vi "HMI.vi"(5 "Disabled?":bool=TRUE, 7 "HMI to Control":T1={"RightDriveValue"=0.0, "LeftDriveValue"=0.0, "Arm Manual "=0.0, "Stacker Manual "=0.0, "Claw Manual "=0.0, "ClawSlightOpenNumber"=0, "Intake Value "=0.0, "Arm States"=enum."4 Tote", "Claw States"=enum."Claw Manual ", "Intake Man. or Sense"=enum."Sensing", "Stacker in Manual?"=FALSE, "Drop Stack? "=FALSE, "Tusk Up Request"=FALSE, "Tusk Down Request"=FALSE, "Inver. Wheels  In Request"=FALSE, "Inverse. Wheels Out Request "=FALSE, "Get Out of Manual Control"=FALSE, "Exit Score State"=FALSE, "DriveStraight Help?"=FALSE, "Stacker Shut Off No."=0, "Stacker Need Off?"=FALSE, "Collecting?"=FALSE, "Go to Hover"=FALSE, "Stack Clamp Lock "=FALSE, "Stack Clamp Unlock "=FALSE, "Claw Intake Value "=0.0, "Stack Clamp Lock No. "=0, "Steal Can (ruin their day?)"=FALSE, "Retract (have mercy?)"=FALSE, "Can Grab No. "=0, "Wench Value to Control "=0.0}, 9 "GamepadData":T5) -> (1 "HMI to Control Out":T1={"RightDriveValue"=0.0, "LeftDriveValue"=0.0, "Arm Manual "=0.0, "Stacker Manual "=0.0, "Claw Manual "=0.0, "ClawSlightOpenNumber"=0, "Intake Value "=0.0, "Arm States"=enum."4 Tote", "Claw States"=enum."Claw Manual ", "Intake Man. or Sense"=enum."Sensing", "Stacker in Manual?"=FALSE, "Drop Stack? "=FALSE, "Tusk Up Request"=FALSE, "Tusk Down Request"=FALSE, "Inver. Wheels  In Request"=FALSE, "Inverse. Wheels Out Request "=FALSE, "Get Out of Manual Control"=FALSE, "Exit Score State"=FALSE, "DriveStraight Help?"=FALSE, "Stacker Shut Off No."=0, "Stacker Need Off?"=FALSE, "Collecting?"=FALSE, "Go to Hover"=FALSE, "Stack Clamp Lock "=FALSE, "Stack Clamp Unlock "=FALSE, "Claw Intake Value "=0.0, "Stack Clamp Lock No. "=0, "Steal Can (ruin their day?)"=FALSE, "Retract (have mercy?)"=FALSE, "Can Grab No. "=0, "Wench Value to Control "=0.0}, 3 "GamepadDataOut":T5)   [LabVIEW 2014]
uses:
  Typedefs/GamepadData.ctl
  Typedefs/HMI_to_Control.ctl
  Typedefs/Arm States.ctl
  Typedefs/ClawStates.ctl
  Typedefs/IntakeWheelSenseOrManual.ctl
  Auton/scriptlib/auto_data.vi
panel:
  in  "Wheel Ramp Step":dbl=1.0 format="%#_13g"
  in  "Throttle Ramp Step":dbl=0.015
  in  "Claw Man Threshold":dbl=0.2
  in  "Throttle Drive Straight Assist Threshold":dbl=0.2
  in  "Wheel Drive Straight Assist Threshold":dbl=0.15
  in  "Man Threshold":dbl=0.3
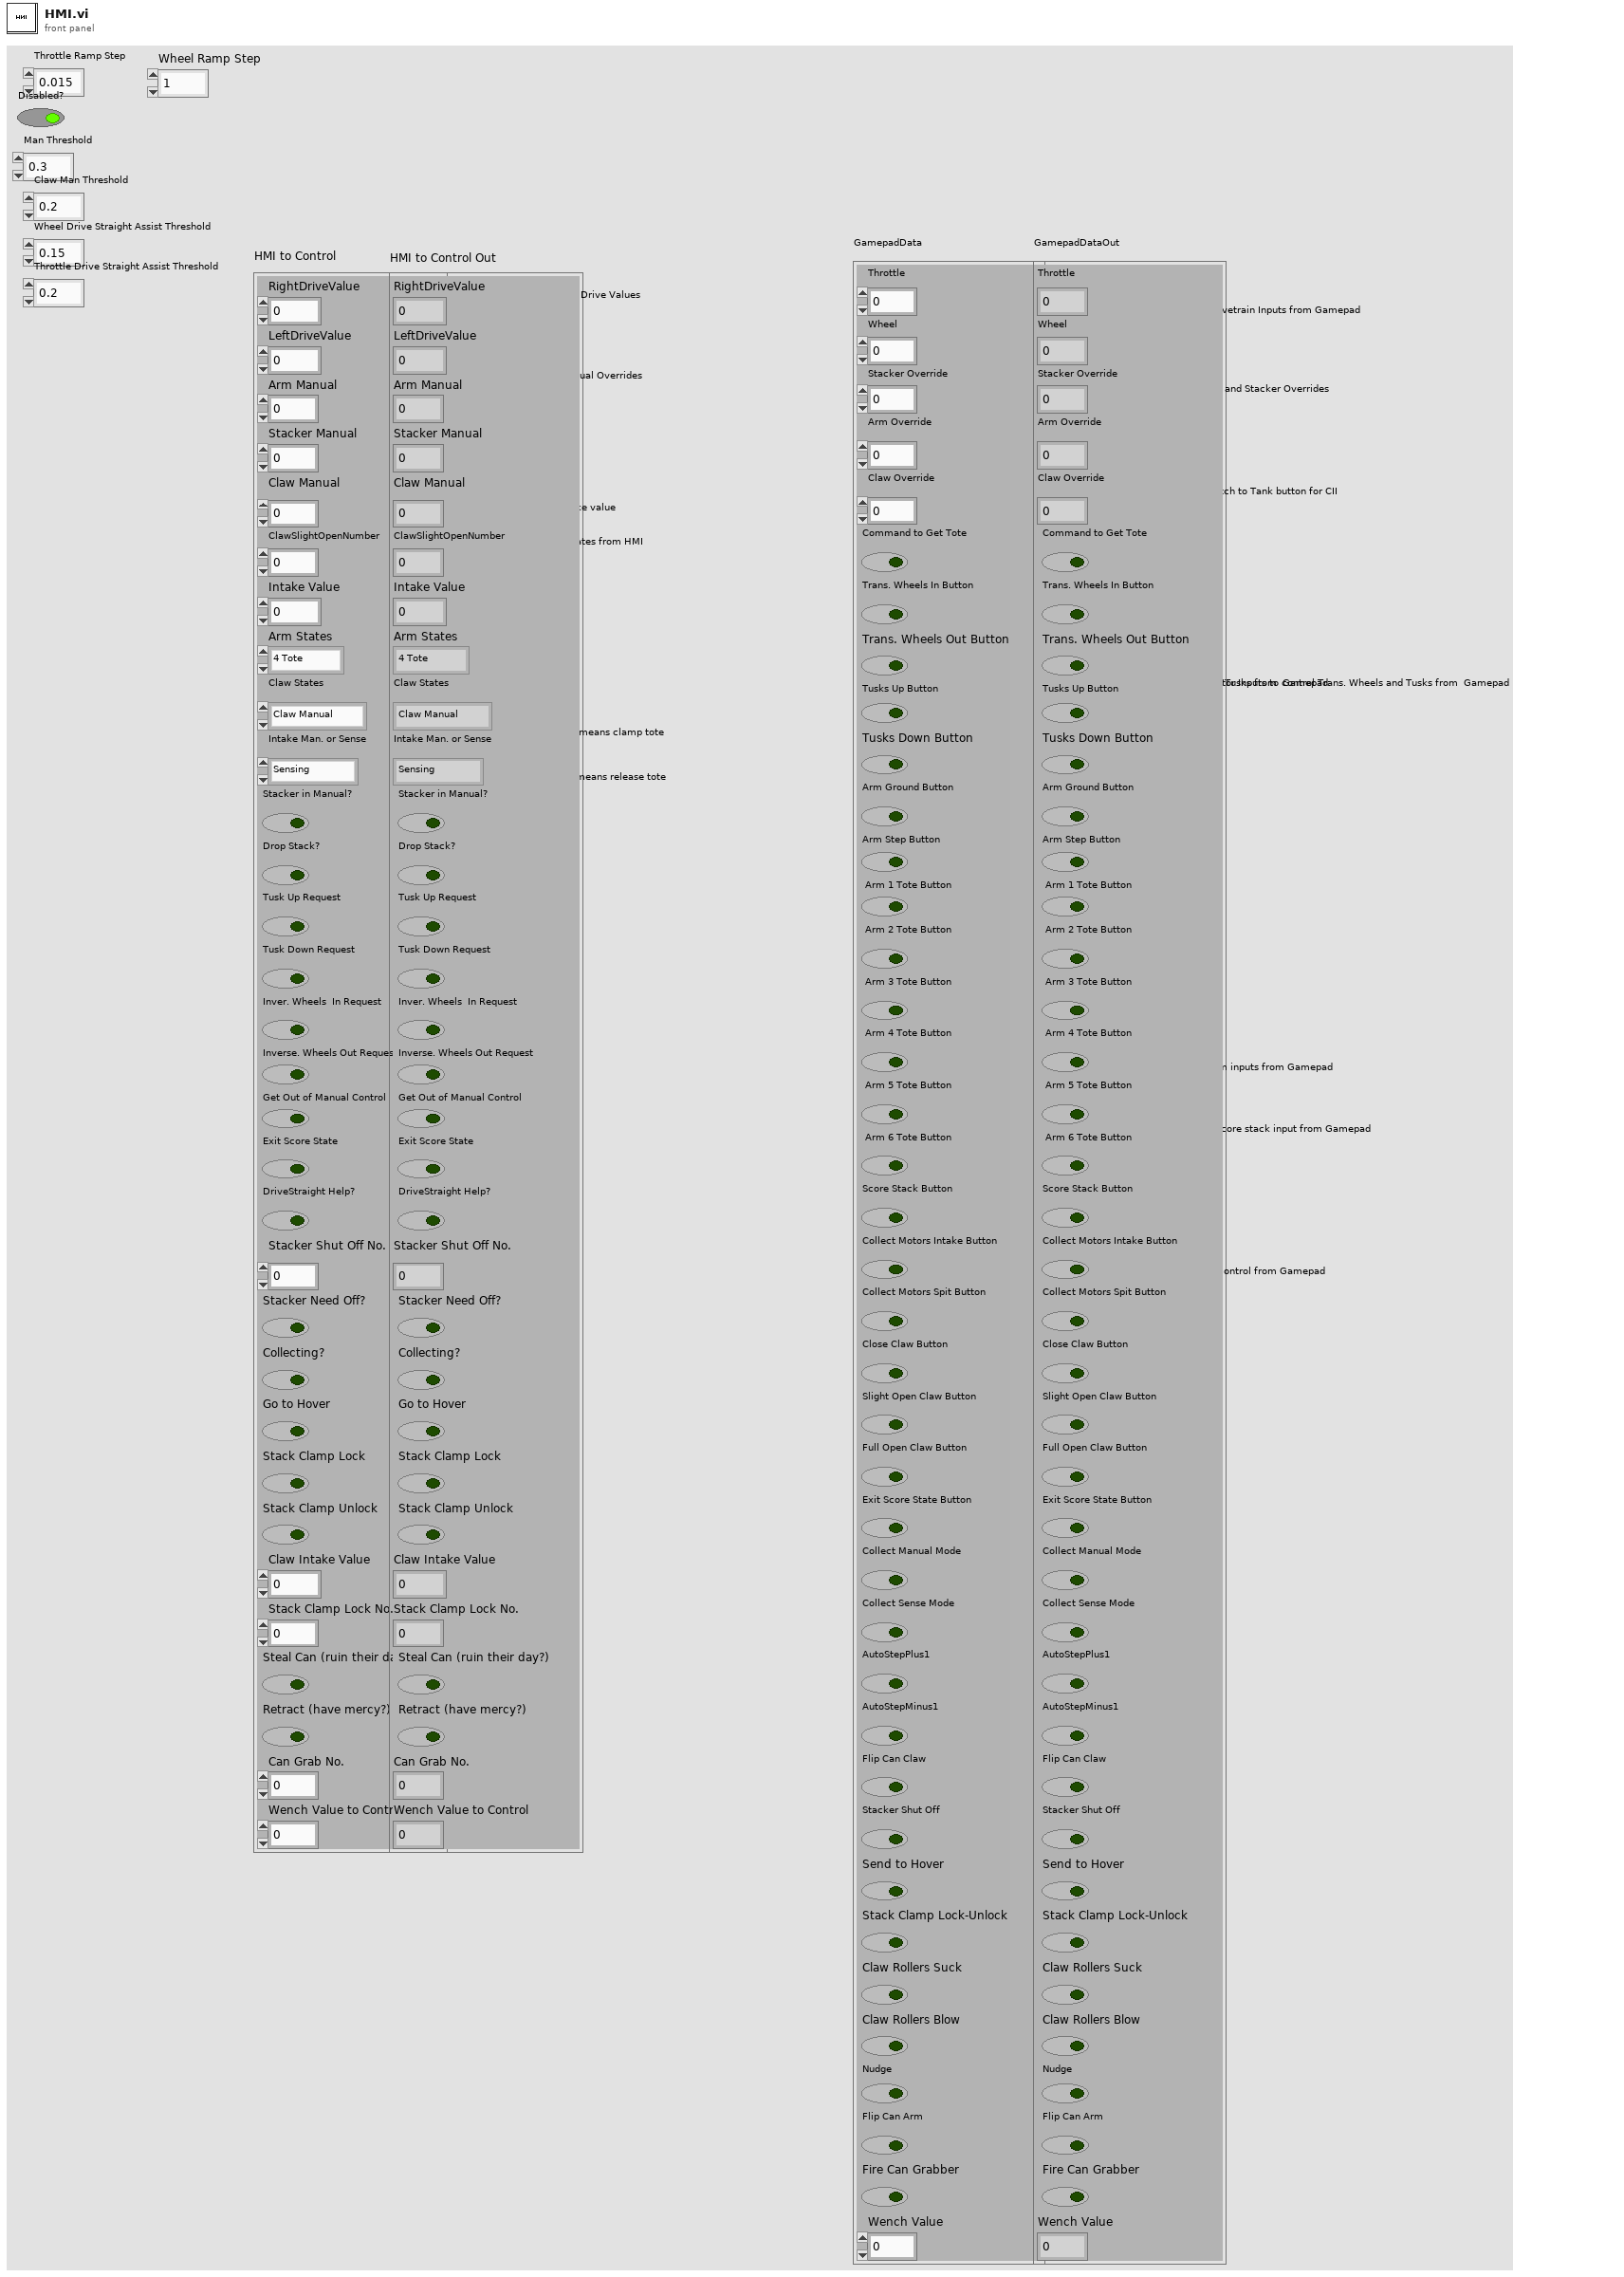
[diagram p1: front panel]
types:
  T1 = typedef "HMI_to_Control.ctl" = cluster{"RightDriveValue":dbl, "LeftDriveValue":dbl, "Arm Manual ":dbl, "Stacker Manual ":dbl, "Claw Manual ":dbl, "ClawSlightOpenNumber":i8, "Intake Value ":sgl, "Arm States":T2, "Claw States":T3, "Intake Man. or Sense":T4, "Stacker in Manual?":bool, "Drop Stack? ":bool, "Tusk Up Request":bool, "Tusk Down Request":bool, "Inver. Wheels  In Request":bool, "Inverse. Wheels Out Request ":bool, "Get Out of Manual Control":bool, "Exit Score State":bool, "DriveStraight Help?":bool, "Stacker Shut Off No.":i8, "Stacker Need Off?":bool, "Collecting?":bool, "Go to Hover":bool, "Stack Clamp Lock ":bool, "Stack Clamp Unlock ":bool, "Claw Intake Value ":sgl, "Stack Clamp Lock No. ":i8, "Steal Can (ruin their day?)":bool, "Retract (have mercy?)":bool, "Can Grab No. ":i8, "Wench Value to Control ":dbl}
  T2 = typedef "Arm States.ctl" = enum16{"Arm Manual ", "Ground", "Step", "1 Tote", "2 Tote", "3 Tote", "4 Tote", "5 Tote", "6 Tote", "Flip Can Arm", "Grab Can in auto", "Nudge"}
  T3 = typedef "ClawStates.ctl" = enum16{"Claw Manual ", "Claw Open", "Claw Closed", "Claw Slight Open", "Flip Can"}
  T4 = typedef "IntakeWheelSenseOrManual.ctl" = enum16{"Sensing", "Manual "}
  T5 = typedef "GamepadData.ctl" = cluster{"Throttle":dbl, "Wheel":dbl, "Stacker Override":dbl, "Arm Override ":dbl, "Claw Override":dbl, "Command to Get Tote":bool, "Trans. Wheels In Button":bool, "Trans. Wheels Out Button":bool, "Tusks Up Button":bool, "Tusks Down Button":bool, "Arm Ground Button":bool, "Arm Step Button":bool, " Arm 1 Tote Button":bool, " Arm 2 Tote Button":bool, " Arm 3 Tote Button ":bool, " Arm 4 Tote Button":bool, " Arm 5 Tote Button":bool, " Arm 6 Tote Button":bool, "Score Stack Button":bool, "Collect Motors Intake Button":bool, "Collect Motors Spit Button":bool, "Close Claw Button":bool, "Slight Open Claw Button":bool, "Full Open Claw Button ":bool, "Exit Score State Button":bool, "Collect Manual Mode ":bool, "Collect Sense Mode":bool, "AutoStepPlus1":bool, "AutoStepMinus1":bool, "Flip Can Claw":bool, "Stacker Shut Off":bool, "Send to Hover ":bool, "Stack Clamp Lock-Unlock ":bool, "Claw Rollers Suck ":bool, "Claw Rollers Blow ":bool, "Nudge":bool, "Flip Can Arm ":bool, "Fire Can Grabber":bool, "Wench Value":dbl}
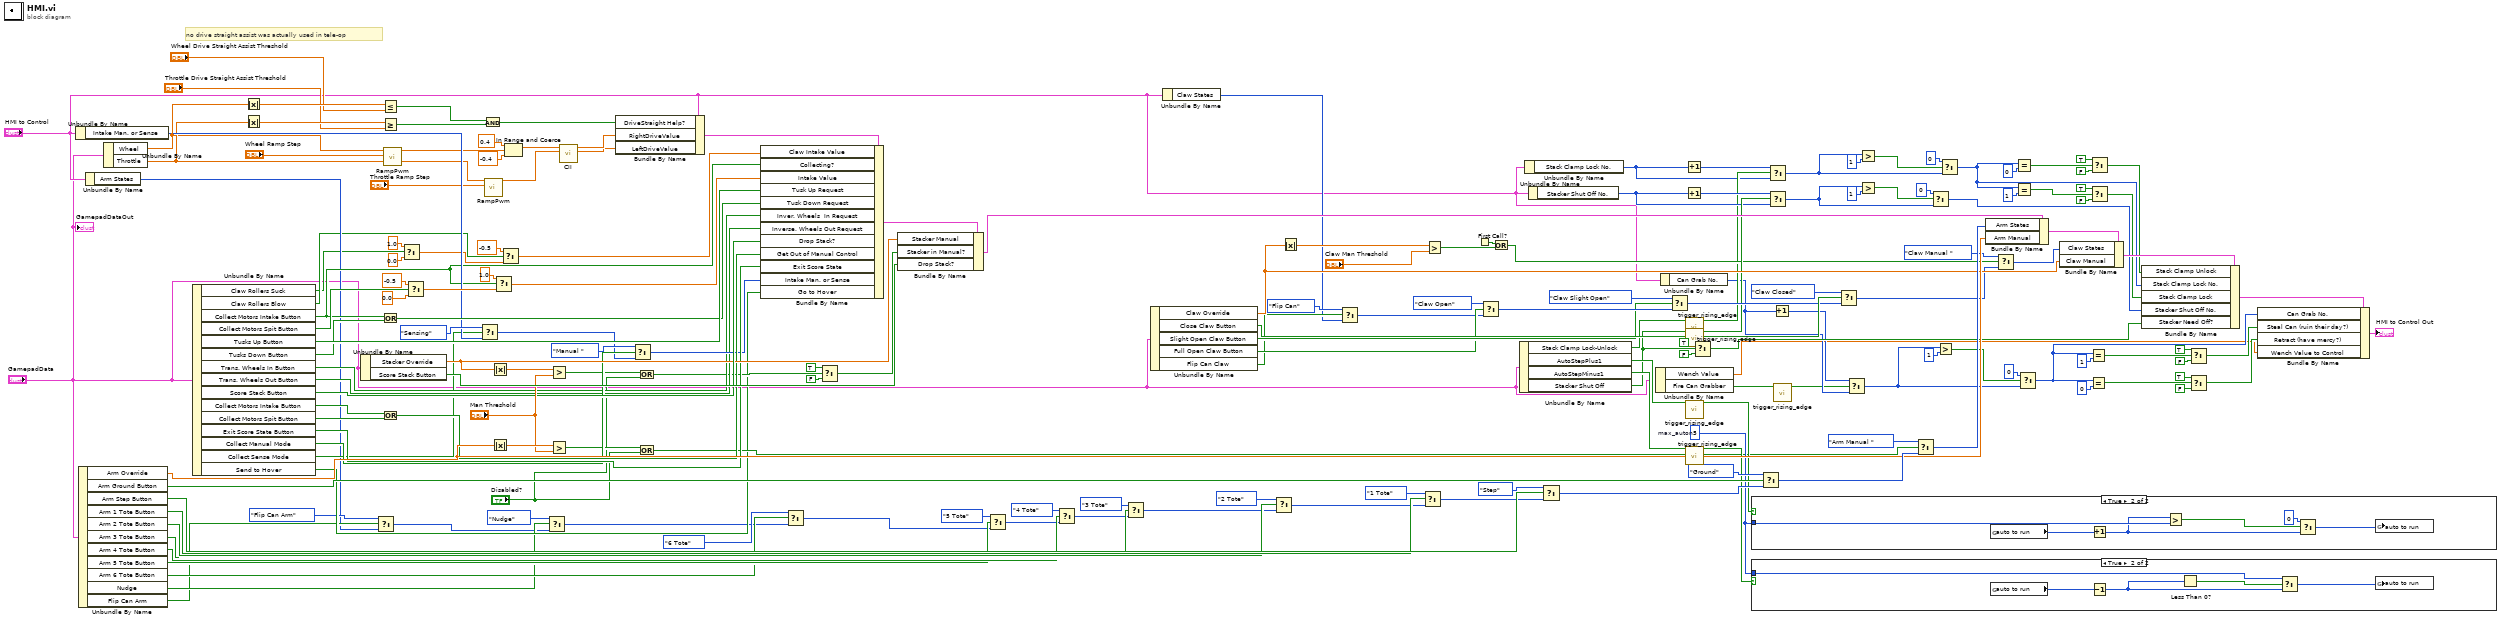
[diagram p0: block diagram]
diagram:
  w90 = i8 5  # max_auton
  # "no drive straight assist was actually used in tele-op"
  n1 = Unbundle By Name("HMI to Control") -> ("Intake Man. or Sense"=w124:T4)
  n2 = Unbundle By Name("GamepadData") -> ("Arm Override"=w148:dbl, "Arm Ground Button"=w174:bool, "Arm Step Button"=w172:bool, "Arm 1 Tote Button"=w170:bool, "Arm 2 Tote Button"=w167:bool, "Arm 3 Tote Button"=w164:bool, "Arm 4 Tote Button"=w161:bool, "Arm 5 Tote Button"=w158:bool, "Arm 6 Tote Button"=w155:bool, "Nudge"=w33:bool, "Flip Can Arm"=w31:bool)
  n3 = Unbundle By Name("HMI to Control") -> ("Arm States"=w30:T2)
  n4 = Unbundle By Name("GamepadData") -> ("Wheel"=w96:dbl, "Throttle"=w98:dbl)
  n5 = Unbundle By Name("GamepadData") -> ("Claw Rollers Suck"=w27:bool, "Claw Rollers Blow"=w28:bool, "Collect Motors Intake Button"=w67:bool, "Collect Motors Spit Button"=w176:bool, "Tusks Up Button"=w132:bool, "Tusks Down Button"=w131:bool, "Trans. Wheels In Button"=w122:bool, "Trans. Wheels Out Button"=w121:bool, "Score Stack Button"=w139:bool, "Collect Motors Intake Button"=w136:bool, "Collect Motors Spit Button"=w135:bool, "Exit Score State Button"=w133:bool, "Collect Manual Mode"=w128:bool, "Collect Sense Mode"=w120:bool, "Send to Hover"=w66:bool)
  n6 = Absolute Value(x=w96) -> (abs(x)=w129:dbl)
  n7 = Absolute Value(x=w98) -> (abs(x)=w118:dbl)
  n8 = Unbundle By Name("GamepadData") -> ("Stacker Override"=w137:dbl, "Score Stack Button"=w147:bool)
  n9 = Select(t=Arm_States."Flip Can Arm" ("Enum"), s=w31, f=w30) -> (s? t:f=w29:T2)
  n10 = Less Or Equal?(x=w129, y="Wheel Drive Straight Assist Threshold") -> (x <= y?=w119:bool)
  n11 = Greater Or Equal?(x=w118, y="Throttle Drive Straight Assist Threshold") -> (x >= y?=w116:bool)
  n12 = Or(x=w67, y=w131) -> (x .or. y?=w130:bool)
  n13 = Or(x=w136, y=w135) -> (x .or. y?=w134:bool)
  n14 = call "RampPwm.vi"("Ramp Step"="Wheel Ramp Step", "Input"=w96) -> ("Output"=w43:dbl)  [unwired: 9 in]
  n15 = Select(t=sgl 1.0, s=w27, f=sgl 0.0) -> (s? t:f=w63:sgl)
  n16 = Select(t=sgl -0.5, s=w176, f=sgl 0.0) -> (s? t:f=w178:sgl)
  n17 = Select(t=IntakeWheelSenseOrManual."Sensing" ("Enum"), s=w120, f=w124) -> (s? t:f=w123:T4)
  n18 = And(x=w119, y=w116) -> (x .and. y?=w115:bool)
  n19 = call "RampPwm.vi"("Ramp Step"="Throttle Ramp Step", "Input"=w98) -> ("Output"=w97:dbl)  [unwired: 9 in]
  n20 = Absolute Value(x=w137) -> (abs(x)=w138:dbl)
  n21 = Absolute Value(x=w148) -> (abs(x)=w152:dbl)
  n22 = Select(t=sgl 1.0, s=w67, f=w178) -> (s? t:f=w141:sgl)
  n23 = Select(t=sgl -0.5, s=w28, f=w63) -> (s? t:f=w65:sgl)
  n24 = In Range and Coerce(upper limit=0.4, x=w43, lower limit=-0.4) -> (coerced(x)=w40:dbl)  [unwired: 1 out]
  n25 = Select(t=Arm_States."Nudge", s=w33, f=w29) -> (s? t:f=w35:T2)
  n26 = Greater?(x=w138, y="Man Threshold") -> (0:w77:bool)
  n27 = Greater?(x=w152, y="Man Threshold") -> (0:w79:bool)
  n28 = call "CII.vi"("Wheel"=w40, "Throttle"=w97) -> ("RightDrive"=w183:dbl, "LeftDrive"=w182:dbl)  [unwired: 7 in]
  n29 = Bundle By Name(cluster="HMI to Control", "DriveStraight Help?"=w115, "RightDriveValue"=w183, "LeftDriveValue"=w182) -> (w181:T1)
  n30 = Select(t=IntakeWheelSenseOrManual."Manual " ("Enum"), s=w128, f=w123) -> (s? t:f=w126:T4)
  n31 = Or(x=w77, y="Disabled?") -> (x .or. y?=w76:bool)
  n32 = Or(x=w79, y="Disabled?") -> (x .or. y?=w78:bool)
  n33 = Bundle By Name(cluster=w181, "Claw Intake Value"=w65, "Collecting?"=w67, "Intake Value"=w141, "Tusk Up Request"=w132, "Tusk Down Request"=w130, "Inver. Wheels  In Request"=w122, "Inverse. Wheels Out Request"=w121, "Drop Stack?"=w139, "Get Out of Manual Control"=w134, "Exit Score State"=w133, "Intake Man. or Sense"=w126, "Go to Hover"=w66) -> (w140:T1)
  n34 = Select(t=Arm_States."6 Tote" ("Enum"), s=w155, f=w35) -> (s? t:f=w153:T2)
  n35 = Select(t=TRUE ("Score Stack Button"), s=w76, f=FALSE ("Score Stack Button")) -> (s? t:f=w143:bool)
  n36 = Bundle By Name(cluster=w140, "Stacker Manual"=w137, "Stacker in Manual?"=w143, "Drop Stack?"=w147) -> (w142:T1)
  n37 = Select(t=Arm_States."5 Tote" ("Enum"), s=w158, f=w153) -> (s? t:f=w156:T2)
  n38 = Select(t=Arm_States."4 Tote" ("Enum"), s=w161, f=w156) -> (s? t:f=w160:T2)
  n39 = Select(t=Arm_States."3 Tote" ("Enum"), s=w164, f=w160) -> (s? t:f=w162:T2)
  n40 = Unbundle By Name("GamepadData") -> ("Claw Override"=w112:dbl, "Close Claw Button"=w106:bool, "Slight Open Claw Button"=w100:bool, "Full Open Claw Button"=w99:bool, "Flip Can Claw"=w38:bool)
  n41 = Unbundle By Name("HMI to Control") -> ("Claw States"=w37:T3)
  n42 = Select(t=Arm_States."2 Tote" ("Enum"), s=w167, f=w162) -> (s? t:f=w165:T2)
  n43 = Absolute Value(x=w112) -> (abs(x)=w111:dbl)
  n44 = Select(t=ClawStates."Flip Can" ("Claw States"), s=w38, f=w37) -> (s? t:f=w36:T3)
  n45 = Select(t=Arm_States."1 Tote" ("Enum"), s=w170, f=w165) -> (s? t:f=w168:T2)
  n46 = Greater?(x=w111, y="Claw Man Threshold") -> (0:w70:bool)
  n47 = First Call?() -> (First Call?: T/F=w68:bool)
  n48 = Select(t=ClawStates."Claw Open" ("Claw States"), s=w99, f=w36) -> (s? t:f=w103:T3)
  n49 = Or(x=w68, y=w70) -> (x .or. y?=w69:bool)
  n50 = Unbundle By Name("GamepadData") -> ("Stack Clamp Lock-Unlock"=w59:bool, "AutoStepPlus1"=w93:bool, "AutoStepMinus1"=w92:bool, "Stacker Shut Off"=w75:bool)
  n51 = Unbundle By Name("HMI to Control") -> ("Stack Clamp Lock No."=w56:i8)
  n52 = Unbundle By Name("HMI to Control") -> ("Stacker Shut Off No."=w85:i8)
  n53 = Select(t=Arm_States."Step" ("Enum"), s=w172, f=w168) -> (s? t:f=w171:T2)
  n54 = Unbundle By Name("GamepadData") -> ("Wench Value"=w1:dbl, "Fire Can Grabber"=w16:bool)
  n55 = Unbundle By Name("HMI to Control") -> ("Can Grab No."=w18:i8)
  n56 = Select(t=ClawStates."Claw Slight Open" ("Claw States"), s=w100, f=w103) -> (s? t:f=w102:T3)
  n57 = Increment(x=w56) -> (x+1=w58:i8)
  n58 = Increment(x=w85) -> (x+1=w86:i8)
  n59 = call "trigger_rising_edge.vi"("input"=w59) -> ("rising"=w57:bool)  [unwired: 10 in]
  n60 = call "trigger_rising_edge.vi"("input"=w75) -> ("rising"=w87:bool)  [unwired: 10 in]
  n61 = call "trigger_rising_edge.vi"("input"=w93) -> ("rising"=w91:bool)  [unwired: 10 in]
  n62 = call "trigger_rising_edge.vi"("input"=w92) -> ("rising"=w89:bool)  [unwired: 10 in]
  n63 = Select(t=TRUE, s=w75, f=FALSE) -> (s? t:f=w72:bool)
  n64 = case shown="True" w91 {
    tunnel: w90 -> [_ w187]
    frame False {
    }
    frame True {
      n65 = global read "auto_data.vi" "auto to run"() -> (w189:i8)
      n66 = Increment(x=w189) -> (x+1=w186:i8)
      n67 = Greater?(x=w186, y=w187) -> (0:w188:bool)
      n68 = Select(t=i8 0, s=w188, f=w186) -> (s? t:f=w184:i8)
      n69 = global write "auto_data.vi" "auto to run"(w184) -> ()
    }
  }
  n70 = case shown="True" w89 {
    tunnel: w90 -> [_ w191]
    frame False {
    }
    frame True {
      n71 = global read "auto_data.vi" "auto to run"() -> (w194:i8)
      n72 = Decrement(x=w194) -> (x-1=w190:i8)
      n73 = Less Than 0?(x=w190) -> (x < 0?=w193:bool)
      n74 = Select(t=w191, s=w193, f=w190) -> (s? t:f=w192:i8)
      n75 = global write "auto_data.vi" "auto to run"(w192) -> ()
    }
  }
  n76 = Select(t=Arm_States."Ground" ("Enum"), s=w174, f=w171) -> (s? t:f=w150:T2)
  n77 = Select(t=w58, s=w57, f=w56) -> (s? t:f=w55:i8)
  n78 = Select(t=w86, s=w87, f=w85) -> (s? t:f=w80:i8)
  n79 = Increment(x=w18) -> (x+1=w20:i8)
  n80 = call "trigger_rising_edge.vi"("input"=w16) -> ("rising"=w15:bool)  [unwired: 10 in]
  n81 = Select(t=ClawStates."Claw Closed" ("Claw States"), s=w106, f=w102) -> (s? t:f=w107:T3)
  n82 = Select(t=w20, s=w15, f=w18) -> (s? t:f=w19:i8)
  n83 = Greater?(x=w55, y=i8 1) -> (0:w61:bool)
  n84 = Greater?(x=w80, y=i8 1) -> (0:w83:bool)
  n85 = Select(t=Arm_States."Arm Manual " ("Enum"), s=w78, f=w150) -> (s? t:f=w149:T2)
  n86 = Select(t=i8 0, s=w83, f=w80) -> (s? t:f=w81:i8)
  n87 = Greater?(x=w19, y=i8 1) -> (0:w22:bool)
  n88 = Select(t=i8 0, s=w61, f=w55) -> (s? t:f=w47:i8)
  n89 = Bundle By Name(cluster=w142, "Arm States"=w149, "Arm Manual"=w148) -> (w113:T1)
  n90 = Select(t=ClawStates."Claw Manual " ("Claw States"), s=w69, f=w107) -> (s? t:f=w101:T3)
  n91 = Equal?(x=w47, y=i8 0) -> (x = y?=w45:bool)
  n92 = Equal?(x=w47, y=i8 1) -> (x = y?=w53:bool)
  n93 = Select(t=i8 0, s=w22, f=w19) -> (s? t:f=w4:i8)
  n94 = Bundle By Name(cluster=w113, "Claw States"=w101, "Claw Manual"=w112) -> (w88:T1)
  n95 = Equal?(x=w4, y=i8 1) -> (x = y?=w11:bool)
  n96 = Equal?(x=w4, y=i8 0) -> (x = y?=w5:bool)
  n97 = Select(t=TRUE, s=w45, f=FALSE) -> (s? t:f=w44:bool)
  n98 = Select(t=TRUE, s=w53, f=FALSE) -> (s? t:f=w50:bool)
  n99 = Bundle By Name(cluster=w88, "Stack Clamp Unlock"=w44, "Stack Clamp Lock No."=w47, "Stack Clamp Lock"=w50, "Stacker Shut Off No."=w81, "Stacker Need Off?"=w72) -> (w14:T1)
  n100 = Select(t=TRUE, s=w11, f=FALSE) -> (s? t:f=w3:bool)
  n101 = Select(t=TRUE, s=w5, f=FALSE) -> (s? t:f=w2:bool)
  n102 = Bundle By Name(cluster=w14, "Can Grab No."=w4, "Steal Can (ruin their day?)"=w3, "Retract (have mercy?)"=w2, "Wench Value to Control"=w1) -> (→"HMI to Control Out":T1)
  "GamepadDataOut" <- "GamepadData"
